vi "Page_Source_Update_On_Add_to_Top.vi"(8 "error in (no error)":errorcluster, 10 "AB_Source in":refnum<class "AB_Source.lvclass">, 11 "AB_RESTfulWebService in":refnum<class "AB_RESTfulWebService.lvclass">) -> (0 "error out":errorcluster, 2 "updated":bool, 3 "AB_RESTfulWebService out":refnum<class "AB_RESTfulWebService.lvclass">)   [LabVIEW 2020, in "AB_RESTfulWebService.lvclass"]
uses:
  <vilib>/AppBuilder/AB_Classes/RESTful/AB_RESTfulWebService.lvclass
  <vilib>/AppBuilder/AB_Classes/Source/AB_Source.lvclass
  <vilib>/AppBuilder/AB_Classes/Source/RESTfulVI/AB_Source_RESTfulVI.lvclass
  e:/builds/penguin/labview/branches/2020/dev/dist/vi.lib/AppBuilder/AB_Classes/Source/AB_Source.lvclass
  <vilib>/AppBuilder/AB_Classes/RESTful/AB_RESTfulWebService.lvclass/AB_RESTfulWebService.ctl
  <vilib>/AppBuilder/AB_Classes/RESTful/AB_RESTful_RoutingTemplate.ctl
  <vilib>/AppBuilder/AB_Classes/RESTful/AB_RESTful_RoutingType.ctl
  <vilib>/AppBuilder/AB_Classes/RESTful/AB_RESTful_HTTPMethodType.ctl
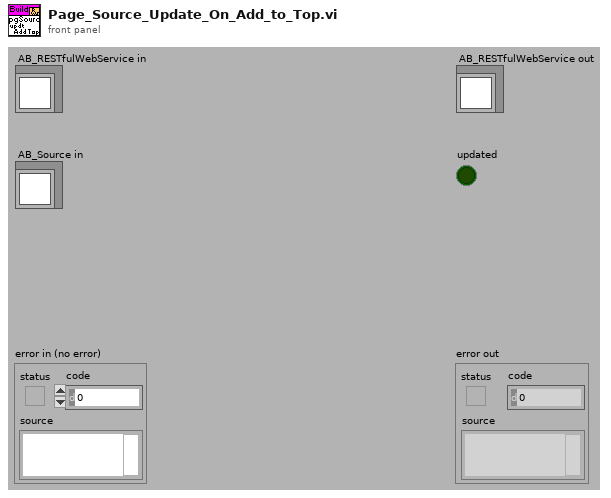
[diagram p1: front panel]
types:
  T1 = typedef "AB_RESTful_RoutingTemplate.ctl" = cluster{"Template":string, "Routing Type":T2, "HTTP Method Type":T3, "VIName":string, "Default String":string, "Require API key":bool, "Auth permissions":string[], "eng_Static Alias":string, "Required Privilege":string}
  T2 = typedef "AB_RESTful_RoutingType.ctl" = enum32{"Method", "Static"}
  T3 = typedef "AB_RESTful_HTTPMethodType.ctl" = enum32{"GET", "POST", "PUT", "DELETE"}
  T4 = typedef "AB_RESTful_Configuration.ctl" = cluster{"Service VI Type":T5, "Load VI at statup":bool, "Keep VI in memory":bool, "Output type":T6, "Output format":T7, "Use headers":bool, "Buffered":bool, "eng_Load VI by name":bool}
  T5 = typedef "AB_RESTful_VIType.ctl" = enum32{"Web Method", "Auxiliary", "eng_Internal", "eng_Content"}
  T6 = typedef "AB_RESTful_OutputType.ctl" = enum32{"Terminal", "Stream"}
  T7 = typedef "AB_RESTful_OutputFormat.ctl" = enum32{"XML", "Text", "HTML", "JSON"}
  T8 = typedef "AB_Source.ctl" = cluster{"path":path, "itemID":string, "parentIndex":i32, "sourceInclusion":T9, "destinationIndex":i32, "properties":T10[], "newName":string, "lvfile":bool, "valid":bool, "eng_inBuild":bool, "eng_isNonVILink":bool, "Amalgamation":bool, "Amalgamation Piece":bool, "eng_delimitedName":string, "preventRename":bool}
  T9 = typedef "AB_Source_Inclusion.ctl" = enum16{"IncludeIfReferenced", "Include", "Exclude", "TopLevel"}
  T10 = typedef "AB_Source_Properties.ctl" = cluster{"sourcePropertyType":T11, "value":variant}
  T11 = typedef "AB_Source_Property_Type.ctl" = enum16{"Remove block diagram", "Remove front panel", "Password", "Window has title bar", "Show menu bar", "Show vertical scroll bar", "Show horizontal scroll bar", "Show toolbar", "Show Abort button", "Show fp when called", "Window behavior", "Allow user to close window", "Window run-time position", "Run when opened", "Allow debugging", "Auto error handling", "Generate guard code", "Use stack variables", "Expression folding", "Integer only", "Inline subVI"}
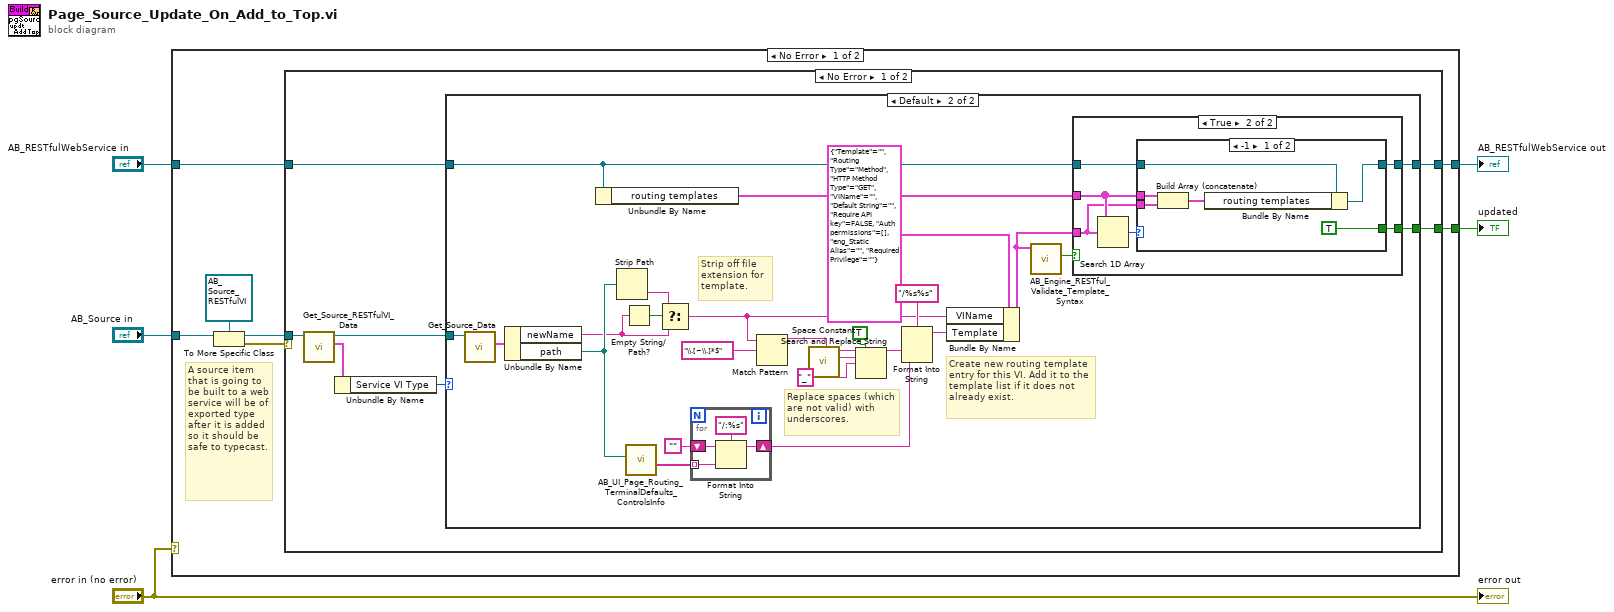
[diagram p0: block diagram]
diagram:
  n1 = case shown="No Error" "error in (no error)" {
    tunnel: "AB_Source in" -> [w9 _]
    tunnel: "AB_RESTfulWebService in" -> [w12 w65]
    tunnel: [w11 w65] -> w3
    tunnel: [w10 _] -> w1
    frame No Error {
      # "A source item that is going to be built to a web service will be of exported type after it is added so it should be safe to typecast."
      n2 = To More Specific Class(target class=refnum<class "AB_Source_RESTfulVI.lvclass"> refnum ("AB_Source_RESTfulVI.lvclass"), reference=w9) -> (specific class reference=w6:refnum<class "AB_Source_RESTfulVI.lvclass">, error out=w7:errorcluster)  [unwired: 1 in]
      n3 = case shown="No Error" w7 {
        tunnel: w12 -> [w19 w64]
        tunnel: [w18 w64] -> w11
        tunnel: [w17 _] -> w10
        tunnel: w6 -> [w16 _]
        frame No Error {
          n4 = call <vilib>:"Get_Source_RESTfulVI_Data.vi"("Class in"=w16) -> ("RESTful VI configuration"=w14:T4, "Class out"=w15:refnum<class "AB_Source_RESTfulVI.lvclass">)  [unwired: 8 in, 1 out]
          n5 = Unbundle By Name(w14) -> ("Service VI Type"=w13:T5)
          n6 = case shown="Default" w13 {
            tunnel: w19 -> [w20 w31]
            tunnel: [w20 w30] -> w18
            tunnel: [_ w29] -> w17
            tunnel: w15 -> [_ w21]
            frame "Auxiliary" {
              # "Do not create default URL maps for aux VIs."
            }
            frame Default {
              # "Replace spaces (which are not valid) with underscores."
              # "Create new routing template entry for this VI. Add it to the template list if it does not already exist."
              # "Strip off file extension for template."
              n7 = call <vilib>:"Get_Source_Data.vi"("Class in"=w21) -> ("data"=w45:T8)  [unwired: 1 in, 9 out]
              n8 = Unbundle By Name(w45) -> ("newName"=w35:string, "path"=w36:path)
              n9 = Unbundle By Name(w31) -> ("routing templates"=w38:T1[])
              n10 = Strip Path(path=w36) -> (name=w34:string)  [unwired: 1 out]
              n11 = Empty String/Path?(string/path=w35) -> (empty?=w37:bool)
              n12 = call <resource>:"AB_UI_Page_Routing_TerminalDefaults_ControlsInfo.vi"("VI path"=w36) -> ("terminal names"=w42:string[])  [unwired: 1 in, 9 out]
              n13 = Select(t=w34, s=w37, f=w35) -> (s? t:f=w32:string)
              n14 = for {
                tunnel: w42 -> [w60] mode=indexing
                shift-right: [w61] -> w44
                shift-left: "" -> [w63]
                n15 = Format Into String(format string="/:%s", initial string=w63, w60) -> (resulting string=w61:string)  [unwired: 1 in, 1 out]
              }
              n16 = Match Pattern(string=w32, regular expression="\\.[~\\.]*$") -> (before substring=w25:string)  [unwired: 4 out]
              n17 = call <vilib>:"Space Constant.vi"() -> ("String"=w27:string)
              n18 = Search and Replace String(replace all?=TRUE ("replace all? (F)"), input string=w25, search string=w27, replace string="_") -> (result string=w24:string)  [unwired: 1 in, 6 out]
              n19 = Format Into String(format string="/%s%s", w24, w44) -> (resulting string=w39:string)  [unwired: 2 in, 1 out]
              n20 = Bundle By Name(cluster=T1 {"Template"="", "Routing Type"=enum."Method", "HTTP Method Type"=enum."GET", "VIName"="", "Default String"="", "Require API key"=FALSE, "Auth permissions"=[], "eng_Static Alias"="", "Required Privilege"=""} ("RESTful VI routing template"), "VIName"=w32, "Template"=w39) -> (w23:T1)
              n21 = call <vilib>:"AB_Engine_RESTful_Validate_Template_Syntax.vi"("RESTful VI routing template in"=w23) -> ("valid syntax"=w22:bool)  [unwired: 10 out]
              n22 = case shown="True" w22 {
                tunnel: w38 -> [_ w51]
                tunnel: w31 -> [w46 w50]
                tunnel: [w46 w49] -> w30
                tunnel: [_ w48] -> w29
                tunnel: w23 -> [_ w47]
                frame False {
                  # "If template syntax is not valid, don't add the default URL map to the list."
                }
                frame True {
                  n23 = Search 1D Array(1D array=w51, element=w47) -> (index of element=w52:i32)  [unwired: 1 out]
                  n24 = case shown="-1" w52 {
                    tunnel: w50 -> [w55 w59]
                    tunnel: [w54 w59] -> w49
                    tunnel: w51 -> [w58 _]
                    tunnel: w47 -> [w57 _]
                    tunnel: [TRUE _] -> w48
                    frame -1 {
                      n25 = Build Array (concatenate)(w58, w57) -> (w56:T1[])
                      n26 = Bundle By Name(cluster=w55, "routing templates"=w56) -> (w54:refnum<class "AB_RESTfulWebService.lvclass">)
                    }
                    frame Default {
                    }
                  }
                }
              }
            }
          }
        }
        frame Error {
          # "Don't do anything in case the source type is not a RESTful VI type."
        }
      }
    }
    frame Error {
    }
  }
  "AB_RESTfulWebService out" <- w3
  "updated" <- w1
  "error out" <- "error in (no error)"
